vi "flattenPressureToXML_Array.vi"(8 "error in (no error)":errorcluster, 9 "pressureUnitInXML":T1, 10 "pressureAgain":variant, 11 "pressure":dbl[unit][](array[numeric])) -> (0 "error out":errorcluster, 3 "xmlString":string)   [LabVIEW 2012, in "UnitsAndXML.lvlib"]
uses:
  <userlib>/Common/UnitsAndXML/UnitsAndXML.lvlib
  <userlib>/Common/UnitsAndXML/FlattenItemWithUnitToXML/FlattenPressureToXML/PressureUnit.ctl
  <vilib>/Utility/VariantDataType/VariantType.lvlib
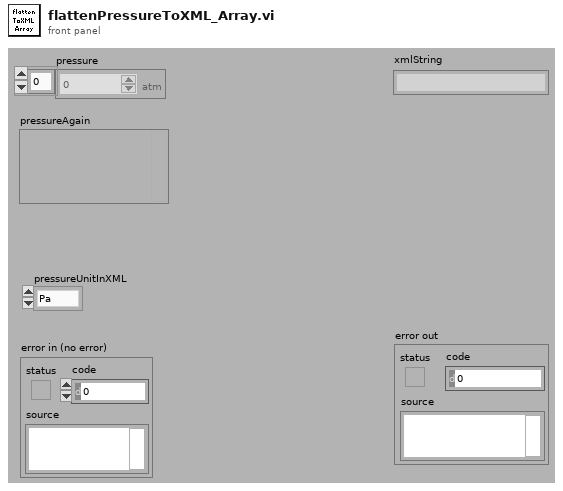
[diagram p1: front panel]
types:
  T1 = typedef "UnitsAndXML.lvlib/PressureUnit.ctl" = enum16{"Pa", "atm", "bar", "mbar", "m.Hg", "psi", "torr"}
  T2 = typedef "VariantType.lvlib/Type.ctl" = enum8{"Invalid Type", "Void", "I8", "I16", "I32", "I64", "U8", "U16", "U32", "U64", "Single Float", "Double Float", "Extended Float", "Single Complex", "Double Complex", "Extended Complex", "Enum U8", "Enum U16", "Enum U32", "Enum U64", "Single Float With Unit", "Double Float With Unit", "Extended Float With Unit", "Single Complex with Unit", "Double Complex with Unit", "Extended Complex with Unit", "Boolean", "String", "Path", "Picture", "Tag", "Array", "Cluster", "Variant", "LV Variant", "Waveform", "Timestamp", "Digital Waveform", "Digital Data", "ExpressData", "Refnum", "External Data", "VI", "Poly VI", "LabVIEW Class Instance", "Fixed Point"}
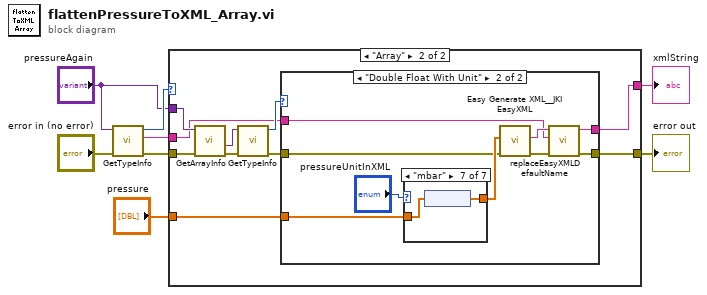
[diagram p0: block diagram]
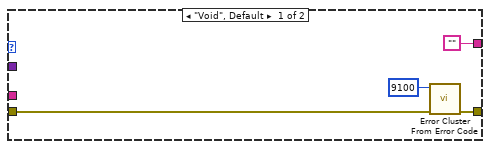
[diagram p2: hidden frame]
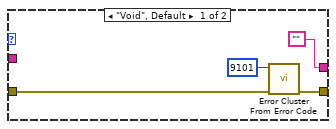
[diagram p3: hidden frame]
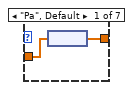
[diagram p4: hidden frame]
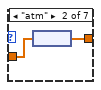
[diagram p5: hidden frame]
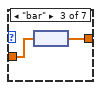
[diagram p6: hidden frame]
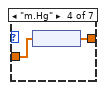
[diagram p7: hidden frame]
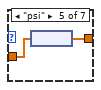
[diagram p8: hidden frame]
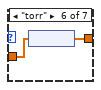
[diagram p9: hidden frame]
diagram:
  n1 = call <vilib>:"GetTypeInfo.vi"("error in (no error)"="error in (no error)", "Variant"="pressureAgain") -> ("error out"=w2:errorcluster, "Name"=w1:string, "Type Enum"=w4:T2)  [unwired: 5 in, 2 out]
  n2 = case shown="\"Array\"" w4 {
    tunnel: "pressure" -> [_ w18]
    tunnel: ["" w16] -> w7
    tunnel: [w9 w17] -> w6
    tunnel: "pressureAgain" -> [_ w22]
    tunnel: w2 -> [w10 w15]
    tunnel: w1 -> [_ w13]
    frame "Void", Default {
      n3 = call <vilib>:"Error Cluster From Error Code.vi"("error in (no error)"=w10, "error code (0)"=9100) -> ("error out"=w9:errorcluster)  [unwired: 7 in]
    }
    frame "Array" {
      n4 = call <vilib>:"GetArrayInfo.vi"("error in (no error)"=w15, "Variant"=w22) -> ("error out"=w21:errorcluster, "ArrayElement"=w20:variant)  [unwired: 6 in, 2 out]
      n5 = call <vilib>:"GetTypeInfo.vi"("error in (no error)"=w21, "Variant"=w20) -> ("error out"=w14:errorcluster, "Type Enum"=w19:T2)  [unwired: 5 in, 3 out]
      n6 = case shown="\"Double Float With Unit\"" w19 {
        tunnel: w18 -> [_ w35]
        tunnel: ["" w32] -> w16
        tunnel: [w23 w30] -> w17
        tunnel: w14 -> [w24 w29]
        tunnel: w13 -> [_ w27]
        frame "Void", Default {
          n7 = call <vilib>:"Error Cluster From Error Code.vi"("error in (no error)"=w24, "error code (0)"=9101) -> ("error out"=w23:errorcluster)  [unwired: 7 in]
        }
        frame "Double Float With Unit" {
          n8 = case shown="\"mbar\"" "pressureUnitInXML" {
            tunnel: w35 -> [w37 w39 w41 w43 w45 w47 w49]
            tunnel: [w36 w38 w40 w42 w44 w46 w48] -> w31
            frame "Pa", Default {
              n9 = node(w37) -> (w36:dbl[])
            }
            frame "atm" {
              n10 = node(w39) -> (w38:dbl[])
            }
            frame "bar" {
              n11 = node(w41) -> (w40:dbl[])
            }
            frame "m.Hg" {
              n12 = node(w43) -> (w42:dbl[])
            }
            frame "psi" {
              n13 = node(w45) -> (w44:dbl[])
            }
            frame "torr" {
              n14 = node(w47) -> (w46:dbl[])
            }
            frame "mbar" {
              n15 = node(w49) -> (w48:dbl[])
            }
          }
          n16 = call <vilib>:"Easy Generate XML__JKI EasyXML.vi"("error in (no error)"=w29, "LabVIEW Data"=w31) -> ("error out"=w28:errorcluster, "XML String"=w33:string)  [unwired: 8 in]
          n17 = call <userlib>:"replaceEasyXMLDefaultName.vi"("error in"=w28, "desiredName"=w27, "easyXMLStringWithDefaultNames"=w33) -> ("error out"=w30:errorcluster, "xmlString"=w32:string)  [unwired: 7 in]
        }
      }
    }
  }
  "xmlString" <- w7
  "error out" <- w6
